vi "Complex A x B (Optimized).vi"(2 "B":T1, 3 "A":T1) -> (0 "error":i32, 1 "A x B":T1)   [LabVIEW 2018, in "NI_AALBase.lvlib"]
uses:
  NI_AALBase.lvlib
  ComplexMatrix.ctl
  <resource>/lvanlys.dll
  NI_Matrix.lvlib
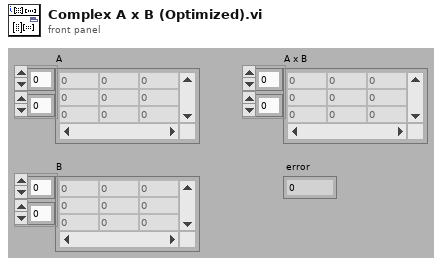
[diagram p1: front panel]
types:
  T1 = typedef "NI_Matrix.lvlib/ComplexMatrix.ctl" = cdb[][]
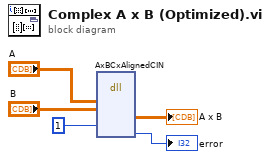
[diagram p0: block diagram]
diagram:
  n1 = dll-call lib="C:/Program Files (x86)/National Instruments/LabVIEW 2018/resource/lvanlys.*" fn="AxBCxAlignedCIN"("aHandle"="A", "bHandle"="B", "isAligned"=1) -> ("A x B"=→"A x B":T1, "dsperr"=→"error":i32)  [unwired: 9 in, 2 out]
